vi "IMUprocess.vi"(9 "Frames Read":u16[](array[numeric]), 11 "error in (no error)":errorcluster) -> (0 "error out":errorcluster, 2 "Gyro deg/s":dbl[](array[numeric]), 3 "Accel g's":dbl[](array[numeric]))   [LabVIEW 2016]
doc: "Inputs\nRaw data from MPU9250\n\nOutputs\nAccelerometer readings\nGyroscope redaings\n\nBitshifts the rawdata and put them in two arrays, one for accelerometer data and for gyroscope data"
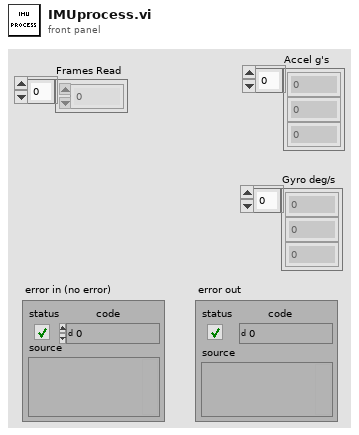
[diagram p1: front panel]
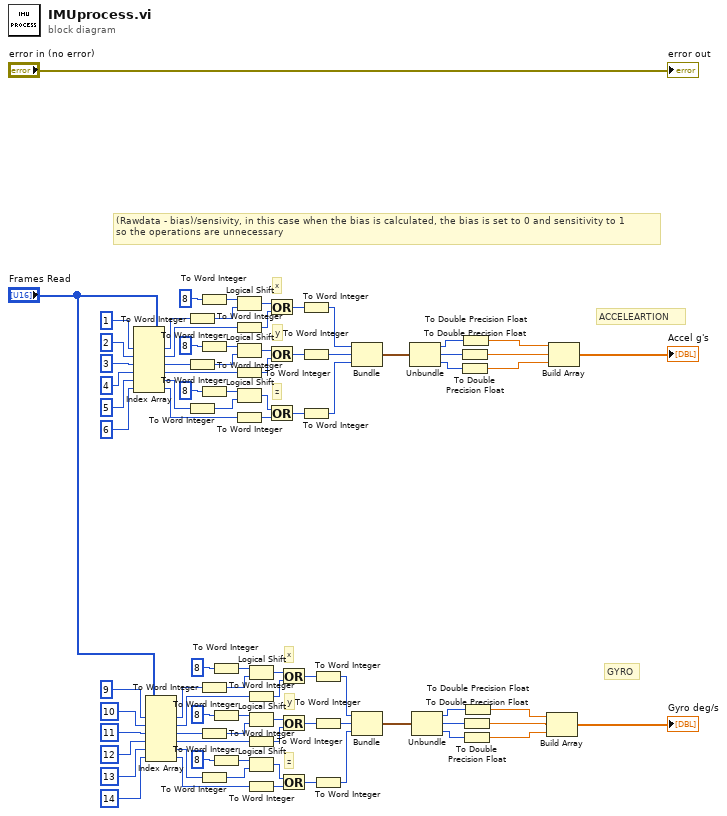
[diagram p0: block diagram]
diagram:
  # "GYRO"
  # "(Rawdata - bias)/sensivity, in this case when the bias is calculated, the bias is set to 0 and sensitivity to 1\nso the operations are unnecessary"
  # "ACCELEARTION"
  # "z"
  # "y"
  # "x"
  # "z"
  # "y"
  # "x"
  n1 = Index Array(array="Frames Read", index #1=1 ("index"), index #2=2 ("index"), index #3=3 ("index"), index #4=4 ("index"), index #5=5 ("index"), index #6=6 ("index")) -> (element #1=w32:u16, element #2=w37:u16, element #3=w45:u16, element #4=w49:u16, element #5=w54:u16, element #6=w55:u16)
  n2 = Index Array(array="Frames Read", index #1=9 ("index"), index #2=10 ("index"), index #3=11 ("index"), index #4=12 ("index"), index #5=13 ("index"), index #6=14 ("index")) -> (element #1=w75:u16, element #2=w76:u16, element #3=w77:u16, element #4=w78:u16, element #5=w79:u16, element #6=w80:u16)
  n3 = To Word Integer(number=w32) -> (16bit integer=w33:i16)
  n4 = To Word Integer(number=w45) -> (16bit integer=w48:i16)
  n5 = To Word Integer(number=w54) -> (16bit integer=w53:i16)
  n6 = To Word Integer(number=i16 8 ("y")) -> (16bit integer=w34:i16)
  n7 = To Word Integer(number=i16 8 ("y")) -> (16bit integer=w47:i16)
  n8 = To Word Integer(number=i16 8 ("y")) -> (16bit integer=w52:i16)
  n9 = To Word Integer(number=w75) -> (16bit integer=w68:i16)
  n10 = To Word Integer(number=w77) -> (16bit integer=w62:i16)
  n11 = To Word Integer(number=w79) -> (16bit integer=w58:i16)
  n12 = To Word Integer(number=i16 8 ("y")) -> (16bit integer=w67:i16)
  n13 = To Word Integer(number=i16 8 ("y")) -> (16bit integer=w63:i16)
  n14 = To Word Integer(number=i16 8 ("y")) -> (16bit integer=w59:i16)
  n15 = Logical Shift(y=w34, x=w33) -> (x << y=w15:i16)
  n16 = To Word Integer(number=w37) -> (16bit integer=w36:i16)
  n17 = Logical Shift(y=w47, x=w48) -> (x << y=w16:i16)
  n18 = To Word Integer(number=w49) -> (16bit integer=w50:i16)
  n19 = Logical Shift(y=w52, x=w53) -> (x << y=w17:i16)
  n20 = To Word Integer(number=w55) -> (16bit integer=w56:i16)
  n21 = Logical Shift(y=w67, x=w68) -> (x << y=w74:i16)
  n22 = To Word Integer(number=w76) -> (16bit integer=w65:i16)
  n23 = Logical Shift(y=w63, x=w62) -> (x << y=w73:i16)
  n24 = To Word Integer(number=w78) -> (16bit integer=w61:i16)
  n25 = Logical Shift(y=w59, x=w58) -> (x << y=w72:i16)
  n26 = To Word Integer(number=w80) -> (16bit integer=w57:i16)
  n27 = Or(x=w15, y=w36) -> (x .or. y?=w26:i16)
  n28 = Or(x=w16, y=w50) -> (x .or. y?=w30:i16)
  n29 = Or(x=w17, y=w56) -> (x .or. y?=w29:i16)
  n30 = Or(x=w74, y=w65) -> (x .or. y?=w71:i16)
  n31 = Or(x=w73, y=w61) -> (x .or. y?=w69:i16)
  n32 = Or(x=w72, y=w57) -> (x .or. y?=w70:i16)
  n33 = To Word Integer(number=w26) -> (16bit integer=w27:i16)
  n34 = To Word Integer(number=w30) -> (16bit integer=w28:i16)
  n35 = To Word Integer(number=w29) -> (16bit integer=w31:i16)
  n36 = To Word Integer(number=w71) -> (16bit integer=w81:i16)
  n37 = To Word Integer(number=w69) -> (16bit integer=w82:i16)
  n38 = To Word Integer(number=w70) -> (16bit integer=w83:i16)
  n39 = Bundle(w27, w28, w31) -> (w25:cluster{i16, i16, i16})  [unwired: 1 in]
  n40 = Bundle(w81, w82, w83) -> (w44:cluster{i16, i16, i16})  [unwired: 1 in]
  n41 = Unbundle(w25) -> (w38:i16, w39:i16, w40:i16)
  n42 = Unbundle(w44) -> (w43:i16, w42:i16, w41:i16)
  n43 = To Double Precision Float(number=w39) -> (double precision float=w7:dbl)
  n44 = To Double Precision Float(number=w40) -> (double precision float=w6:dbl)
  n45 = To Double Precision Float(number=w38) -> (double precision float=w8:dbl)
  n46 = To Double Precision Float(number=w42) -> (double precision float=w3:dbl)
  n47 = To Double Precision Float(number=w41) -> (double precision float=w2:dbl)
  n48 = To Double Precision Float(number=w43) -> (double precision float=w4:dbl)
  n49 = Build Array(w4, w3, w2) -> (→"Gyro deg/s":dbl[])
  n50 = Build Array(w8, w7, w6) -> (→"Accel g's":dbl[])
  "error out" <- "error in (no error)"
